vi "TDTSyn-Get Epochs.vi"(0 "TTankX":refnum<k7>, 1 "Epoch code":string="Tick", 5 "T1":dbl, 7 "T2":dbl, 9 "code":dbl, 11 "error in (no error)":errorcluster, 12 "Max Read":i32=1000) -> (4 "Got 'em all":bool, 6 "Number of epochs":i32, 8 "Epoch times":dbl[][](array[numeric]), 15 "error out":errorcluster)   [LabVIEW 2020]
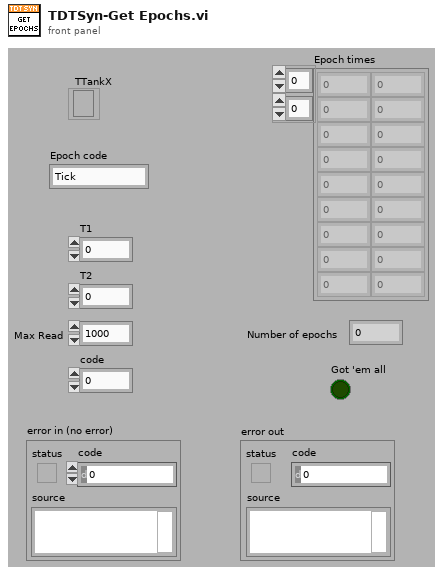
[diagram p1: front panel]
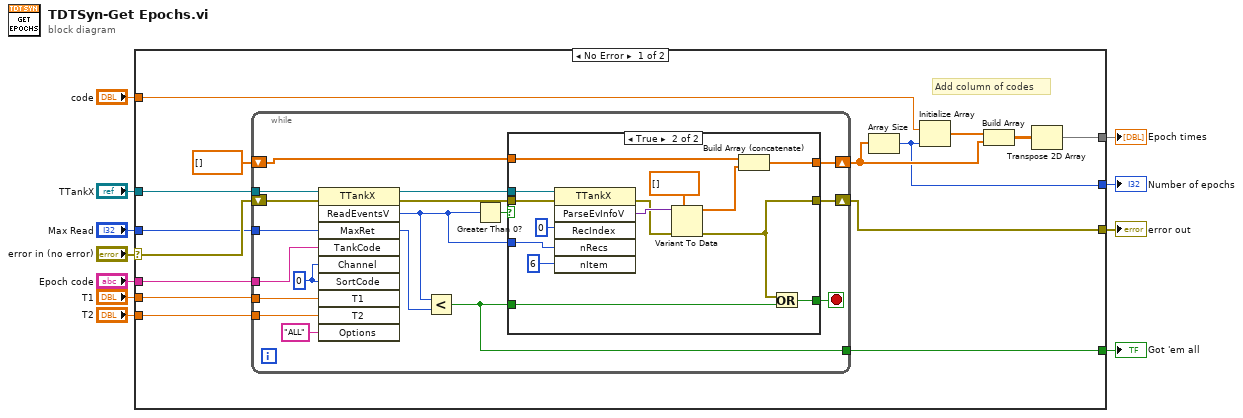
[diagram p0: block diagram]
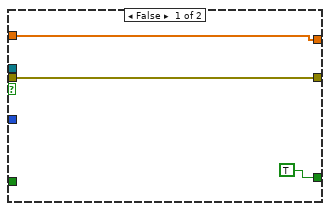
[diagram p2: hidden frame]
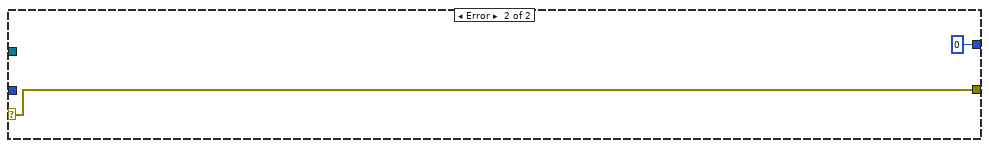
[diagram p3: hidden frame]
diagram:
  n1 = case shown="No Error" "error in (no error)" {
    selector: "error in (no error)" -> [w26 w63]
    tunnel: "Max Read" -> [w25 _]
    tunnel: [w12 w63] -> w9
    tunnel: [w20 _] -> w8
    tunnel: [w19 0] -> w7
    tunnel: "T2" -> [w18 _]
    tunnel: [w17 _] -> w5
    tunnel: "Epoch code" -> [w16 _]
    tunnel: "T1" -> [w15 _]
    tunnel: "TTankX" -> [w14 _]
    tunnel: "code" -> [w13 _]
    frame No Error {
      # "Add column of codes"
      n2 = while {
        tunnel: w14 -> [w44]
        tunnel: w25 -> [w42]
        tunnel: w15 -> [w30]
        shift-right: [w35] -> w22
        shift-left: dbl[] [] -> [w34]
        tunnel: w18 -> [w29]
        tunnel: [w31] -> w17
        tunnel: w16 -> [w28]
        shift-right: [w27] -> w12
        shift-left: w26 -> [w43]
        stop <- w38 stop-if-true
        w40 = 0 ("Channel")
        n3 = invoke class="TTankX" method="ReadEventsV"(reference=w44, error in=w43, "MaxRet"=w42, "TankCode"=w28, "Channel"=w40, "SortCode"=w40, "T1"=w30, "T2"=w29, "Options"="ALL") -> (reference out=w37:refnum<k7>, error out=w36:errorcluster, "ReadEventsV"=w32:i32, "MaxRet"=w39:i32)  [unwired: 1 in, 6 out]
        n4 = Less?(x=w32, y=w39) -> (x < y?=w31:bool)
        n5 = Greater Than 0?(x=w32) -> (x > 0?=w33:bool)
        n6 = case shown="True" w33 {
          tunnel: [TRUE w61] -> w38
          tunnel: w31 -> [_ w60]
          tunnel: w37 -> [_ w59]
          tunnel: w36 -> [w46 w58]
          tunnel: w32 -> [_ w56]
          tunnel: [w47 w50] -> w35
          tunnel: w34 -> [w47 w49]
          tunnel: [w46 w48] -> w27
          frame False {
          }
          frame True {
            n7 = invoke class="TTankX" method="ParseEvInfoV"(reference=w59, error in=w58, "RecIndex"=0, "nRecs"=w56, "nItem"=6) -> (error out=w52:errorcluster, "ParseEvInfoV"=w54:variant)  [unwired: 1 in, 4 out]
            n8 = Variant To Data(error in=w52, type=dbl[] [], Variant=w54) -> (data=w51:dbl[], error out=w48:errorcluster)
            n9 = Build Array (concatenate)(w49, w51) -> (w50:dbl[])
            n10 = Or(x=w48, y=w60) -> (x .or. y?=w61:bool)
          }
        }
      }
      n11 = Array Size(array=w22) -> (size(s)=w19:i32)
      n12 = Initialize Array(w13, w19) -> (w23:dbl[])
      n13 = Build Array(w23, w22) -> (w21:dbl[][])
      n14 = Transpose 2D Array(2D array=w21) -> (transposed array=w20:dbl[][])
    }
    frame Error {
    }
  }
  "Epoch times" <- w8
  "error out" <- w9
  "Number of epochs" <- w7
  "Got 'em all" <- w5
